vi "Sequence.AddVariables.vi"(8 "error in (no error)":errorcluster, 10 "Channels":T1[](array[typedef]), 11 "Sequence":refnum<k24>) -> (0 "error out":errorcluster, 3 "Sequence out":refnum<k24>)   [LabVIEW 2013, in "Simple Sequence Tools - Editor.lvlib"]
uses:
  Simple Sequence Tools - Editor.lvlib
  NationalInstruments.VeriStand.RealTimeSequenceDefinitionApi
  Shared/Types/Channel.Properties.ctl
  Shared/SubVIs/Main.Constants.vi
  Shared/Simple Sequence Tools - Shared.lvlib
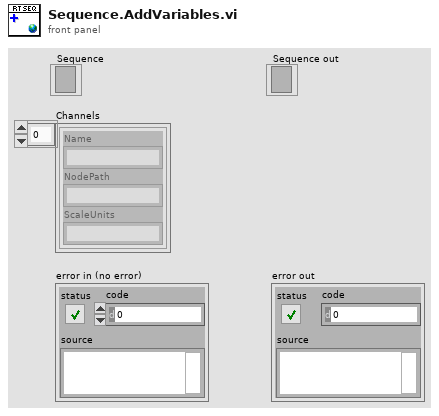
[diagram p1: front panel]
types:
  T1 = typedef "Simple Sequence Tools - Shared.lvlib/Channel.Properties.ctl" = cluster{"Name":string, "NodePath":string, "ScaleUnits":string}
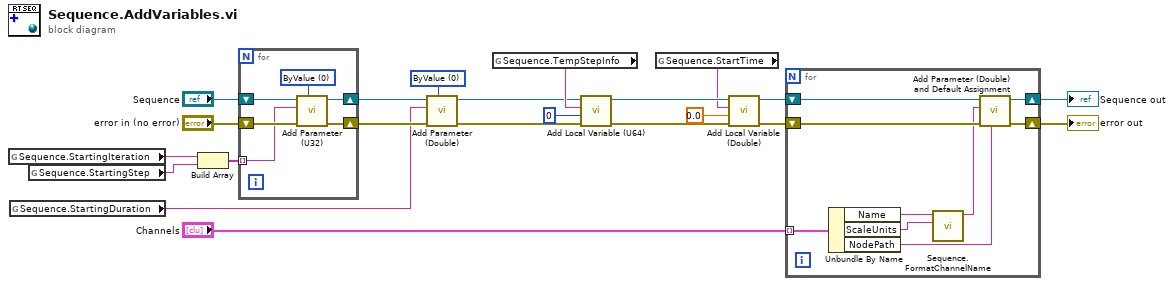
[diagram p0: block diagram]
diagram:
  w6 = 0 items=["ByValue", "ByReference"] ("Evaluation Method (ByReference)")
  n1 = global read "Main.Constants.vi" "Sequence.StartingIteration"() -> (w19:string)
  n2 = global read "Main.Constants.vi" "Sequence.StartingDuration"() -> (w1:string)
  n3 = global read "Main.Constants.vi" "Sequence.StartingStep"() -> (w20:string)
  n4 = Build Array(w19, w20) -> (w21:string[])
  n5 = for {
    shift-right: [w28] -> w4
    shift-left: "error in (no error)" -> [w25]
    shift-right: [w27] -> w5
    shift-left: "Sequence" -> [w26]
    tunnel: w21 -> [w23] mode=indexing
    w24 = 0 items=["ByValue", "ByReference"] ("Evaluation Method (ByReference)")
    n6 = call "Add Parameter (U32).vi"("Evaluation Method (ByReference)"=w24, "error in (no error)"=w25, "Identifier"=w23, "Sequence Ref in"=w26) -> ("error out"=w28:errorcluster, "Sequence Ref out"=w27:refnum<k24>)  [unwired: 6 in]
  }
  n7 = call "Add Parameter (Double).vi"("Evaluation Method (ByReference)"=w6, "error in (no error)"=w4, "Identifier"=w1, "Sequence Ref in"=w5) -> ("error out"=w3:errorcluster, "Sequence Ref out"=w2:refnum<k24>)  [unwired: 6 in]
  n8 = global read "Main.Constants.vi" "Sequence.TempStepInfo"() -> (w22:string)
  n9 = call "Add Local Variable (U64).vi"("error in (no error)"=w3, "Value"=u64 0, "Identifier"=w22, "Sequence Ref in"=w2) -> ("error out"=w8:errorcluster, "Sequence Ref out"=w17:refnum<k24>)  [unwired: 6 in]
  n10 = global read "Main.Constants.vi" "Sequence.StartTime"() -> (w10:string)
  n11 = call "Add Local Variable (Double).vi"("error in (no error)"=w8, "Value"=0.0, "Identifier"=w10, "Sequence Ref in"=w17) -> ("error out"=w7:errorcluster, "Sequence Ref out"=w11:refnum<k24>)  [unwired: 6 in]
  n12 = for {
    tunnel: "Channels" -> [w37] mode=indexing
    shift-right: [w30] -> w13
    shift-left: w7 -> [w33]
    shift-right: [w29] -> w14
    shift-left: w11 -> [w34]
    n13 = Unbundle By Name(w37) -> ("Name"=w36:string, "ScaleUnits"=w35:string, "NodePath"=w31:string)
    n14 = call "Sequence.FormatChannelName.vi"("ScaleUnits"=w35, "Name"=w36) -> ("ChannelName"=w32:string)  [unwired: 9 in]
    n15 = call "Add Parameter (Double) and Default Assignment.vi"("Default Assignment"=w31, "error in (no error)"=w33, "Identifier"=w32, "Sequence Ref in"=w34) -> ("error out"=w30:errorcluster, "Sequence Ref out"=w29:refnum<k24>)  [unwired: 6 in]
  }
  "Sequence out" <- w14
  "error out" <- w13
